vi "AES-InvCipher-text.vi"(5 "Initializer Vector":string, 7 "Operation Mode":T1, 8 "error in (no error)":errorcluster, 10 "Cipher Key":string, 11 "ciphertext":string) -> (0 "error out":errorcluster, 3 "plaintext":string)   [LabVIEW 2010, in "Encryption.lvlib"]
doc: "Decipher a AES-encrypted message using the Cipher key and Operation Mode.\n\nCAUTION:\nThis VI is not secure, it does not protect the memory of the encryption, key and unencrypted data.\n\n(c) Ton Plomp, 2011\nTHIS SOFTWARE IS PROVIDED AS IS, AND ANY WARRANTY IS REJECTED"
uses:
  Encryption.lvlib
  AES-Modes.ctl
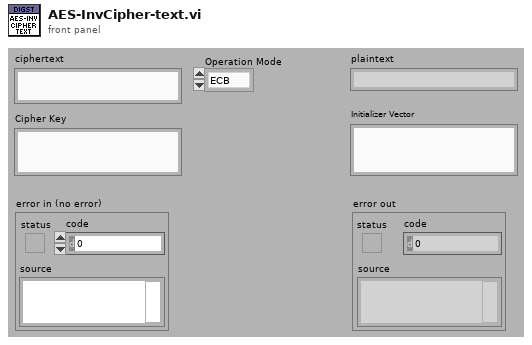
[diagram p1: front panel]
types:
  T1 = typedef "Encryption.lvlib/AES-Modes.ctl" = enum16{"ECB", "CBC", "CFB128", "OFB"}
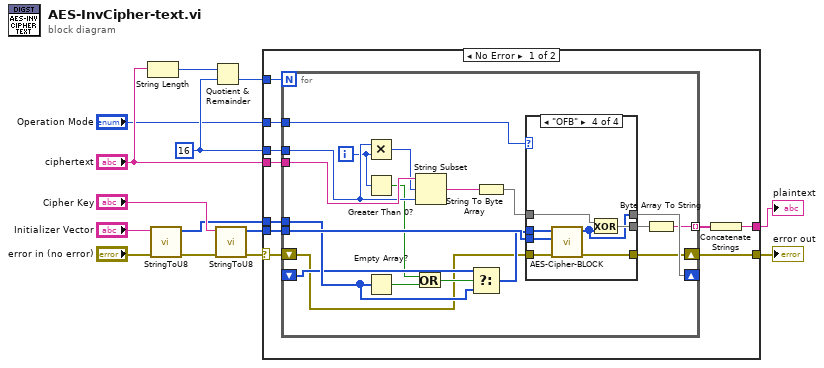
[diagram p0: block diagram]
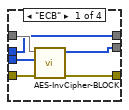
[diagram p2: hidden frame]
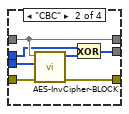
[diagram p3: hidden frame]
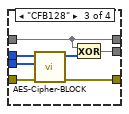
[diagram p4: hidden frame]
diagram:
  w7 = 16 ("y")
  n1 = String Length(string="ciphertext") -> (length=w11:i32)
  n2 = call "StringToU8.vi"("error in (no error)"="error in (no error)", "HEX text in"="Initializer Vector") -> ("error out"=w4:errorcluster, "ArrayU8 out"=w2:u8[])  [unwired: 8 in]
  n3 = Quotient & Remainder(x=w11, y=w7) -> (floor(x/y)=w6:i32)  [unwired: 1 out]
  n4 = call "StringToU8.vi"("error in (no error)"=w4, "HEX text in"="Cipher Key") -> ("error out"=w10:errorcluster, "ArrayU8 out"=w9:u8[])  [unwired: 8 in]
  n5 = case shown="No Error" w10 {
    selector: w10 -> [w20 w71]
    tunnel: "ciphertext" -> [w24 _]
    tunnel: [w19 w71] -> w13
    tunnel: w9 -> [w23 _]
    tunnel: w6 -> [w22 _]
    tunnel: w7 -> [w21 _]
    tunnel: [w17 _] -> w8
    tunnel: w2 -> [w15 _]
    tunnel: "Operation Mode" -> [w16 _]
    frame No Error {
      n6 = for {
        N: w22 -> [_]
        tunnel: w24 -> [w42]
        tunnel: w23 -> [w43]
        tunnel: w21 -> [w40]
        shift-right: [w35] -> w19
        shift-left: w20 -> [w27]
        tunnel: [w37] -> w18 mode=indexing
        shift-right: [w38] -> _
        shift-left: _ -> [w33]
        tunnel: w16 -> [w39]
        tunnel: w15 -> [w34]
        i -> [w31]
        n7 = Multiply(x=w40, y=w31) -> (x*y=w41:i32)
        n8 = Greater Than 0?(x=w31) -> (x > 0?=w30:bool)
        n9 = Empty Array?(array=w34) -> (empty?=w29:bool)
        n10 = Or(x=w30, y=w29) -> (x .or. y?=w28:bool)
        n11 = String Subset(string=w42, offset (0)=w41, length (rest)=w40) -> (substring=w26:string)
        n12 = Select(t=w33, s=w28, f=w34) -> (s? t:f=w32:u8[])
        n13 = String To Byte Array(string=w26) -> (unsigned byte array=w25:u8[])
        n14 = case shown="\"OFB\"" w39 {
          tunnel: w43 -> [w49 w56 w63 w70]
          tunnel: w25 -> [w48 w53 w57 w65]
          tunnel: w27 -> [w47 w55 w62 w69]
          tunnel: [w46 w50 w59 w67] -> w36
          tunnel: [w45 w54 w61 w68] -> w35
          tunnel: w32 -> [w44 w52 w58 w66]
          tunnel: [w44 w53 w57 w64] -> w38
          frame "ECB" {
            n15 = call "AES-InvCipher-BLOCK.vi"("error in (no error)"=w47, "Cipher Key"=w49, "cipher [U8]"=w48) -> ("error out"=w45:errorcluster, "plain [U8]"=w46:u8[])  [unwired: 7 in]
          }
          frame "CBC" {
            n16 = call "AES-InvCipher-BLOCK.vi"("error in (no error)"=w55, "Cipher Key"=w56, "cipher [U8]"=w53) -> ("error out"=w54:errorcluster, "plain [U8]"=w51:u8[])  [unwired: 7 in]
            n17 = Exclusive Or(1:w51, 2:w52) -> (0:w50:u8[])
          }
          frame "CFB128" {
            n18 = call "AES-Cipher-BLOCK.vi"("error in (no error)"=w62, "Cipher Key"=w63, "Plain [U8]"=w58) -> ("error out"=w61:errorcluster, "cipher [U8]"=w60:u8[])  [unwired: 7 in]
            n19 = Exclusive Or(1:w60, 2:w57) -> (0:w59:u8[])
          }
          frame "OFB" {
            n20 = call "AES-Cipher-BLOCK.vi"("error in (no error)"=w69, "Cipher Key"=w70, "Plain [U8]"=w66) -> ("error out"=w68:errorcluster, "cipher [U8]"=w64:u8[])  [unwired: 7 in]
            n21 = Exclusive Or(1:w64, 2:w65) -> (0:w67:u8[])
          }
        }
        n22 = Byte Array To String(unsigned byte array=w36) -> (string=w37:string)
      }
      n23 = Concatenate Strings(w18) -> (w17:string)
    }
    frame Error {
    }
  }
  "error out" <- w13
  "plaintext" <- w8
